vi "Calculate Speed.vi"(1 "radius":dbl, 2 "dimension":dbl, 3 "rotational":dbl, 4 "translational":dbl) -> (0 "speed":dbl)   [LabVIEW 2014]
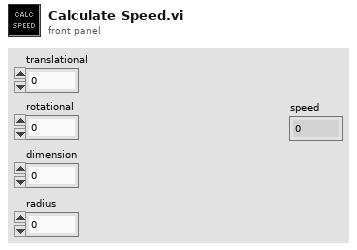
[diagram p1: front panel]
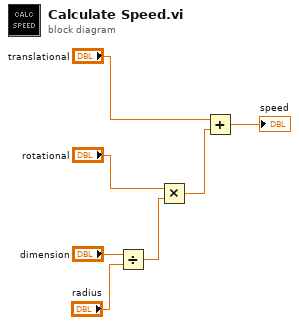
[diagram p0: block diagram]
diagram:
  n1 = Divide(x="dimension", y="radius") -> (x/y=w6:dbl)
  n2 = Multiply(x="rotational", y=w6) -> (x*y=w3:dbl)
  n3 = Add(x="translational", y=w3) -> (x+y=→"speed":dbl)
